vi "GET.comics.upcoming.vi"(4 "series offset":u32, 5 "request specific headers":T3[](array[typedef]), 6 "Number of Series to GET":u32, 7 "timeout (60000)":i32=60000, 8 "error in (no error)":errorcluster, 11 "REST Client in":refnum<class "REST Client.lvclass">) -> (0 "error out":errorcluster, 2 "data":T1, 3 "REST Client out":refnum<class "REST Client.lvclass">)   [LabVIEW 2024]
uses:
  <vilib>/addons/_JKI.lib/REST Client/classes/REST Client/HTTP Header.ctl
  <vilib>/NI/Advanced HTTP Client/Header--Combo Box.ctl
  <vilib>/addons/_JKI.lib/REST Client/classes/REST Client/REST Client.lvclass
  TypeDefs/comics.reply--cluster.ctl
  TypeDefs/comic--cluster.ctl
  <vilib>/NI/Advanced HTTP Client/Session.lvclass
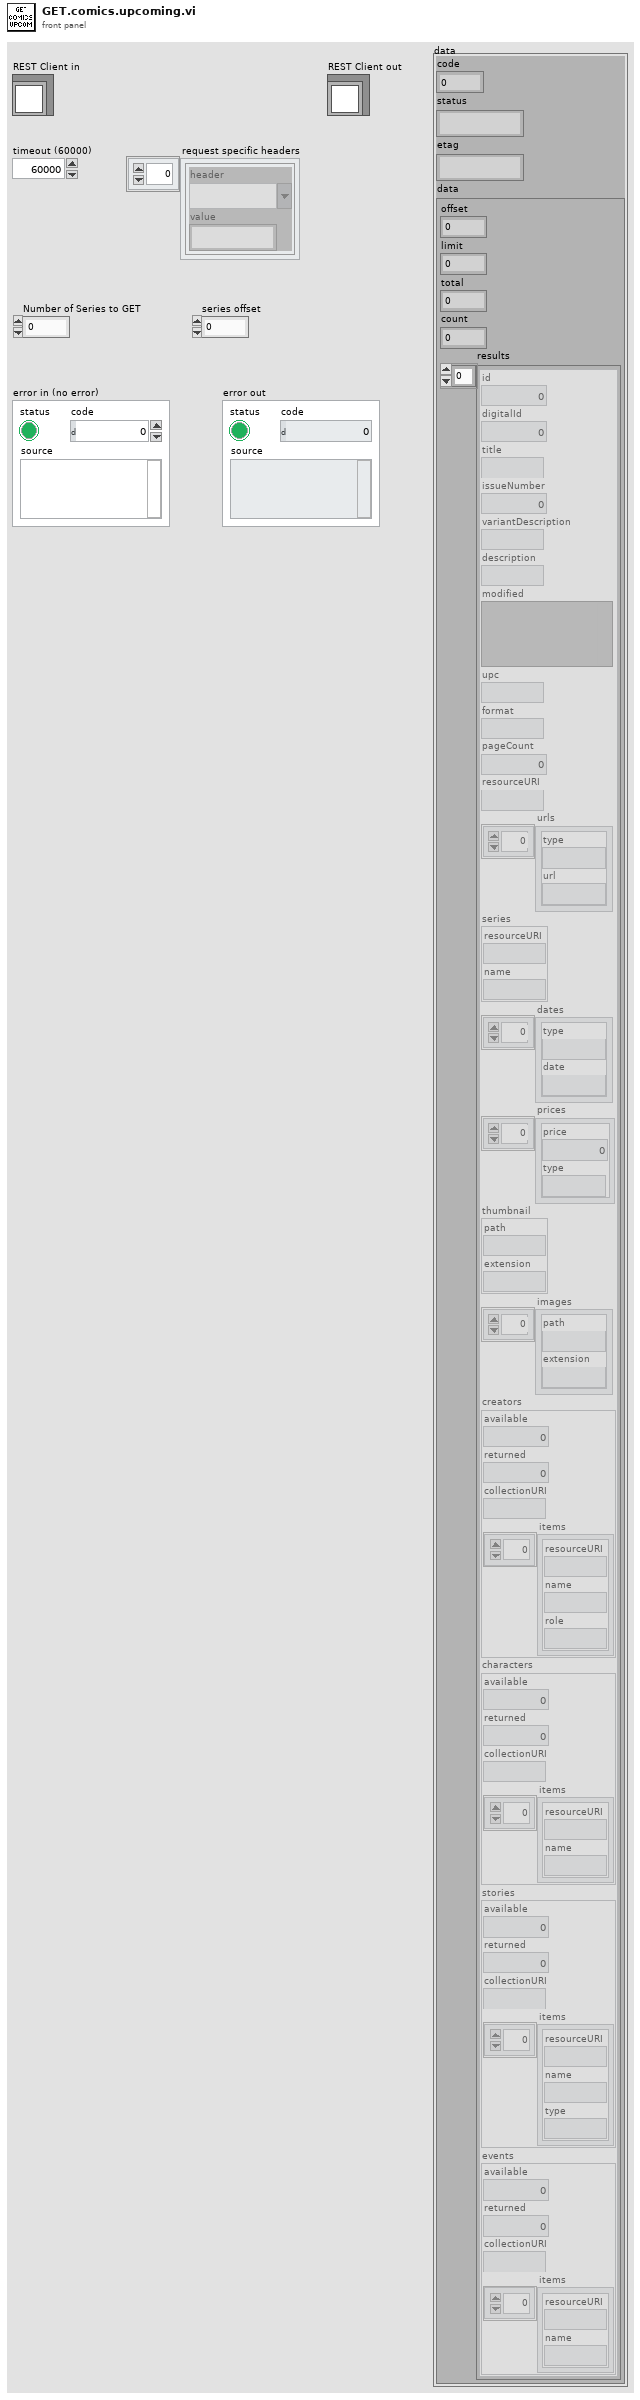
[diagram p1: front panel]
types:
  T1 = typedef "comics.reply--cluster.ctl" = cluster{"code":i32, "status":string, "etag":string, "data":cluster{"offset":i32, "limit":i32, "total":i32, "count":i32, "results":T2[]}}
  T2 = typedef "comic--cluster.ctl" = cluster{"id":i32, "digitalId":i32, "title":string, "issueNumber":i32, "variantDescription":string, "description":string, "modified":variant, "upc":string, "format":string, "pageCount":i32, "resourceURI":string, "urls":cluster{"type":string, "url":string}[], "series":cluster{"resourceURI":string, "name":string}, "dates":cluster{"type":string, "date":string}[], "prices":cluster{"price":dbl, "type":string}[], "thumbnail":cluster{"path":string, "extension":string}, "images":cluster{"path":string, "extension":string}[], "creators":cluster{"available":i32, "returned":i32, "collectionURI":string, "items":cluster{"resourceURI":string, "name":string, "role":string}[]}, "characters":cluster{"available":i32, "returned":i32, "collectionURI":string, "items":cluster{"resourceURI":string, "name":string}[]}, "stories":cluster{"available":i32, "returned":i32, "collectionURI":string, "items":cluster{"resourceURI":string, "name":string, "type":string}[]}, "events":cluster{"available":i32, "returned":i32, "collectionURI":string, "items":cluster{"resourceURI":string, "name":string}[]}}
  T3 = typedef "REST Client.lvlib/REST Client.lvclass/HTTP Header.ctl" = cluster{"header":T4, "value":string}
  T4 = typedef "lib_NI_Advanced HTTP Client.lvlib/Session.lvclass/Header--Combo Box.ctl" = string
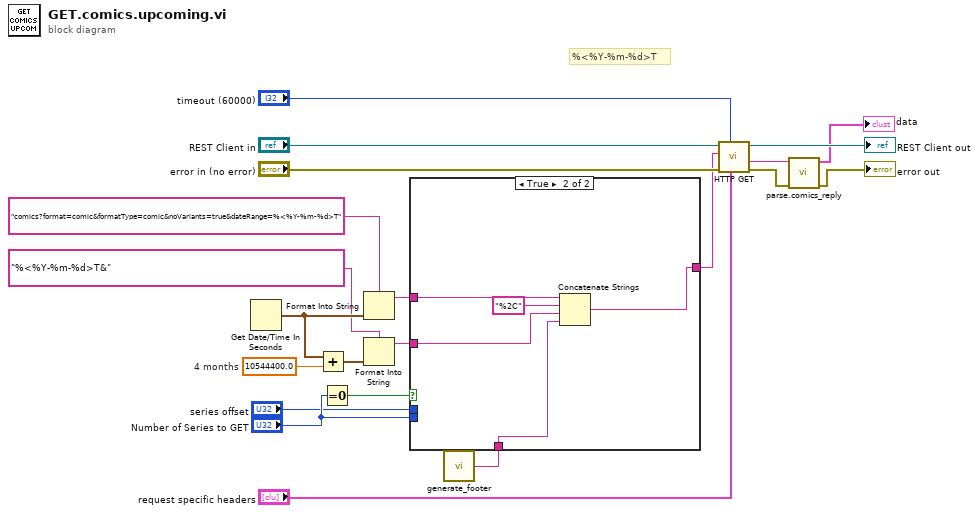
[diagram p0: block diagram]
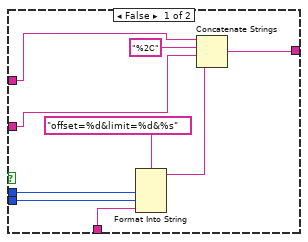
[diagram p2: hidden frame]
diagram:
  w7 = 10544400.0  # 4 months
  # "%<%Y-%m-%d>T"
  n1 = Get Date/Time In Seconds() -> (seconds since 1Jan1904=w8:timestamp)
  n2 = Add(x=w8, y=w7) -> (x+y=w5:timestamp)
  n3 = Equal To 0?(x="Number of Series to GET") -> (x = 0?=w11:bool)
  n4 = Format Into String(format string="comics?format=comic&formatType=comic&noVariants=true&dateRange=%<%Y-%m-%d>T" ("Path"), w8) -> (resulting string=w3:string)  [unwired: 2 in, 1 out]
  n5 = Format Into String(format string="%<%Y-%m-%d>T&" ("Path"), w5) -> (resulting string=w2:string)  [unwired: 2 in, 1 out]
  n6 = call "generate_footer.vi"() -> ("footer"=w17:string)  [unwired: 1 in]
  n7 = case shown="True" w11 {
    tunnel: [w22 w31] -> w1
    tunnel: w17 -> [w30 w32]
    tunnel: "series offset" -> [w29 _]
    tunnel: "Number of Series to GET" -> [w28 _]
    tunnel: w3 -> [w25 w35]
    tunnel: w2 -> [w24 w33]
    frame False {
      n8 = Format Into String(format string="offset=%d&limit=%d&%s" ("Path"), w29, w28, w30) -> (resulting string=w23:string)  [unwired: 2 in, 1 out]
      n9 = Concatenate Strings(w25, "%2C" ("string"), w24, w23) -> (w22:string)
    }
    frame True {
      n10 = Concatenate Strings(w35, "%2C" ("string"), w33, w32) -> (w31:string)
    }
  }
  n11 = call-dynamic "HTTP GET.vi"("request specific headers"="request specific headers", "timeout (0 = Use Default)"="timeout (60000)", "error in (no error)"="error in (no error)", "Path"=w1, "REST Client in"="REST Client in") -> ("error out"=w19:errorcluster, "Response body"=w18:string, "REST Client out"=→"REST Client out":refnum<class "REST Client.lvclass">)  [unwired: 1 in, 3 out]
  n12 = call "parse.comics_reply.vi"("error in"=w19, "string in"=w18) -> ("error out"=→"error out":errorcluster, "data"=→"data":T1)  [unwired: 8 in]
